vi "Value Change.vi"(11 "New Data":variant) -> (3 "Change?":bool)   [LabVIEW 2020]
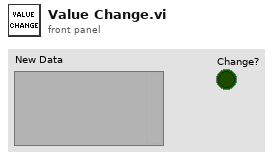
[diagram p1: front panel]
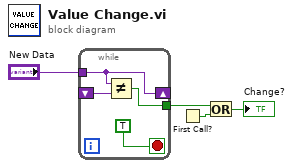
[diagram p0: block diagram]
diagram:
  n1 = while {
    tunnel: "New Data" -> [w8]
    shift-right: [w8] -> _
    shift-left: _ -> [w7]
    tunnel: [w6] -> w3
    stop <- TRUE stop-if-true
    n2 = Not Equal?(x=w8, y=w7) -> (x != y?=w6:bool)
  }
  n3 = First Call?() -> (First Call?: T/F=w2:bool)
  n4 = Or(x=w3, y=w2) -> (x .or. y?=→"Change?":bool)
